vi "fgv_gmap_config.vi"(7 "cmd":enum16{"read", "write"}(ring), 8 "error in":errorcluster, 11 "gmap cfg":T1={"zoom"=16.0, "dt clear"=40, "dt add "=1000, "PinDropMrkr"=enum."red_dot", "zoom n center"=FALSE}) -> (0 "error out":errorcluster, 3 "gmap cfg out":T1={"zoom"=0.0, "dt clear"=0, "dt add "=0, "PinDropMrkr"=enum."red_dot", "zoom n center"=FALSE})   [LabVIEW 2019]
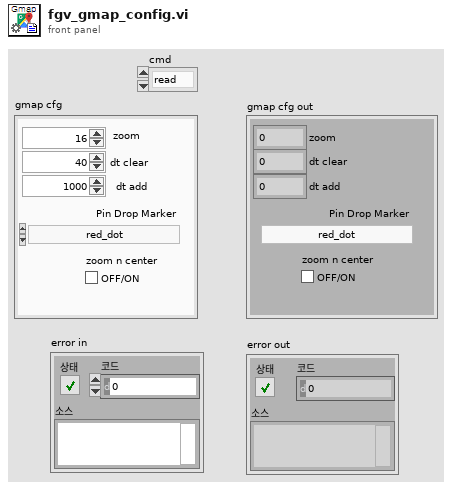
[diagram p1: front panel]
types:
  T1 = cluster{"zoom":dbl, "dt clear":u32, "dt add ":u32, "PinDropMrkr":enum16{"none", "arrow", "blue", "blue_small", "blue_dot", "blue_pushpin", "brown_small", "gray_small", "green", "green_small", "green_dot", "green_pushpin", "green_big_go", "yellow", "yellow_small", "yellow_dot", "yellow_big_pause", "yellow_pushpin", "lightblue", "lightblue_dot", "lightblue_pushpin", "orange", "orange_small", "orange_dot", "pink", "pink_dot", "pink_pushpin", "purple", "purple_small", "purple_dot", "purple_pushpin", "red", "red_small", "red_dot", "red_pushpin", "red_big_stop", "black_small", "white_small"}, "zoom n center":bool}
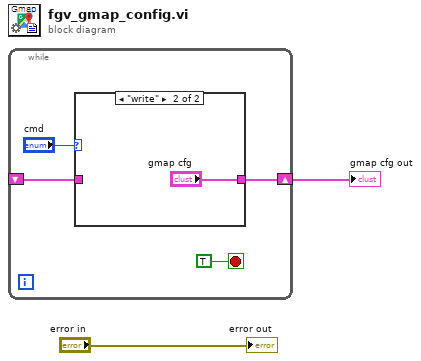
[diagram p0: block diagram]
diagram:
  n1 = while {
    shift-right: [w4] -> w1
    shift-left: _ -> [w3]
    stop <- TRUE stop-if-true
    n2 = case shown="\"write\"" "cmd" {
      tunnel: [w7 "gmap cfg"] -> w4
      tunnel: w3 -> [w7 _]
      frame "read", Default {
      }
      frame "write" {
      }
    }
  }
  "gmap cfg out" <- w1
  "error out" <- "error in"
